vi "All Ring Control Representations.vi"(0 "Ring (Byte)":i8(ring)=3 items=["Value MIN (-128)"=-128, "Value 5"=5, "Value 4"=4, "Value 3"=3, "Value -1"=-1, "Value -2"=-2, "Value MAX (127)"=127], 1 "Ring (Unsigned Byte)":u8(ring)=2 items=["Value MIN (0)"=0, "Value 3"=3, "Value 2"=2, "Value 1"=1, "Value 4"=4, "Value 5"=5, "Value MAX (255)"=255], 2 "Ring (Word)":i16(ring)=32767 items=["Value MIN (-32,768)"=-32768, "Value 1234"=1234, "Value 4578"=4578, "Value -7435"=-7435, "Value -9137"=-9137, "Value -22255"=-22255, "Value MAX (32,767)"=32767], 3 "Ring (Unsigned Word)":u16(ring)=1177 items=["Value MIN (0)"=0, "Value 30000"=30000, "Value 2789"=2789, "Value 1177"=1177, "Value 49999"=49999, "Value 61378"=61378, "Value MAX (65,535)"=65535], 4 "Ring (Long)":i32(ring)=-2147483648 items=["Value MIN (-2,147,483,648)"=-2147483648, "Value -1345781"=-1345781, "Value 392371521"=392371521, "Value 3339955"=3339955, "Value -1137000"=-1137000, "Value -123232"=-123232, "Value MAX (2,147,483,647)"=2147483647], 5 "Ring (Unsigned Long)":u32(ring)=4111777221 items=["Value MIN (0)"=0, "Value 37894532"=37894532, "Value 4111777221"=4111777221, "Value 1"=1, "Value 445"=445, "Value 578901"=578901, "Value MAX (4,294,967,295)"=4294967295], 6 "Ring (Single)":sgl(ring)=3.9 format="%#_13g" items=["Value 1.2"=1.2, "Value 5.7"=5.7, "Value 1.5"=1.5, "Value 3.9"=3.9, "Value 1234.123"=1234.123], 7 "Ring (Quad)  4":i64(ring)=4123456789123456789 items=["Value MIN (-9,223,372,036,854,775,808)"=-9223372036854775808, "Value 51234567890123"=51234567890123, "Value 4123456789123456789"=4123456789123456789, "Value 0"=0, "Value -123456789123456"=-123456789123456, "Value -2456789123456789"=-2456789123456789, "Value MAX (9,223,372,036,854,775,807)"=9223372036854775807], 8 "Ring (Double)":dbl(ring)=5.78 items=["Value 4.57"=4.57, "Value 8.91"=8.91, "Value 5.78"=5.78, "Value 7.23"=7.23], 9 "Ring (Unsigned Quad)":u64(ring)=18446744073709551615 items=["Value MIN (0)"=0, "Value 31234567891259746"=31234567891259746, "Value 21597864123578942"=21597864123578942, "Value 8"=8, "Value 41597534682"=41597534682, "Value 51236974568"=51236974568, "Value MAX (18,446,744,073,709,551,615)"=18446744073709551615], 10 "Ring (Extended)":ext(ring)=44.0 items=["Value 11", "Value 22", "Value 33", "Value 44"]) -> ()   [LabVIEW 2012]
panel:
  in  "stop":bool
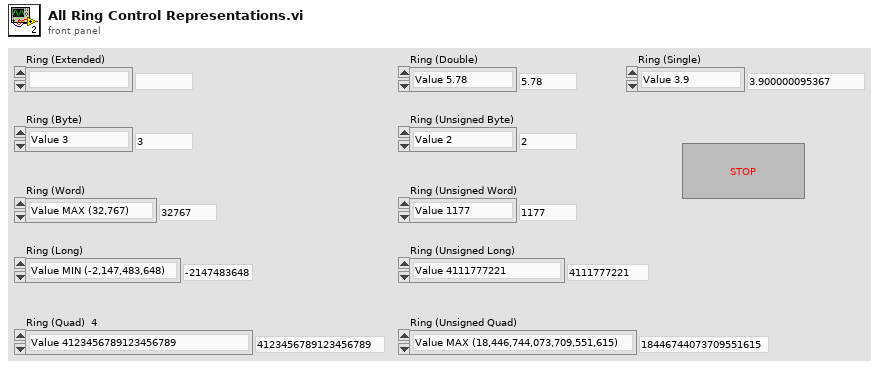
[diagram p1: front panel]
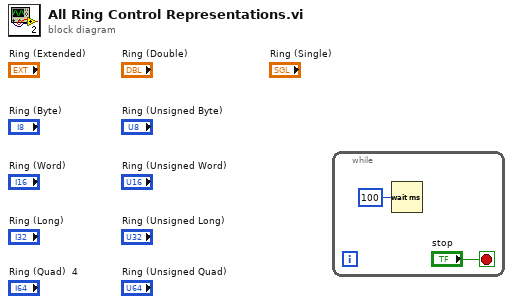
[diagram p0: block diagram]
diagram:
  n1 = while {
    stop <- "stop" stop-if-true
    n2 = Wait (ms)(milliseconds to wait=u32 100) -> ()  [unwired: 1 out]
  }
